vi "Parse Time.vi"(7 "Time In":T1, 10 "Time Index":i32, 11 "Fields In":string[](array[string])) -> (3 "Fields":string[](array[string]), 5 "Time":T1)   [LabVIEW 2012, in "nmea.lvlib" / "nmea.lvclass"]
uses:
  nmea.lvclass
  <vilib>/Utility/miscctls.llb/LVDateTimeRec.ctl
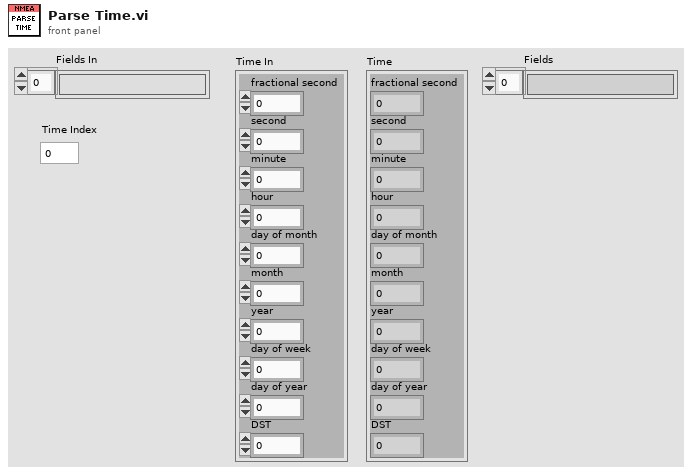
[diagram p1: front panel]
types:
  T1 = typedef "LVDateTimeRec.ctl" = cluster{"fractional second":dbl, "second":i32, "minute":i32, "hour":i32, "day of month":i32, "month":i32, "year":i32, "day of week":i32, "day of year":i32, "DST":i32}
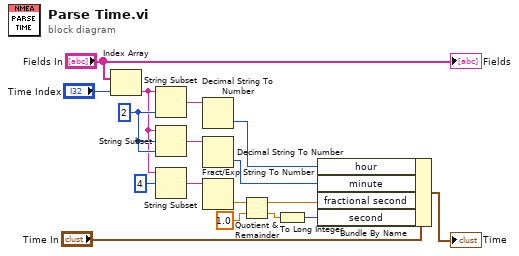
[diagram p0: block diagram]
diagram:
  w16 = 2 ("length (rest)")
  n1 = Index Array(array="Fields In", index="Time Index") -> (element=w15:string)
  n2 = String Subset(string=w15, length (rest)=w16) -> (substring=w11:string)  [unwired: 1 in]
  n3 = String Subset(string=w15, offset (0)=w16, length (rest)=w16) -> (substring=w12:string)
  n4 = String Subset(string=w15, offset (0)=4) -> (substring=w13:string)  [unwired: 1 in]
  n5 = Decimal String To Number(string=w11) -> (number=w2:i32)  [unwired: 2 in, 1 out]
  n6 = Decimal String To Number(string=w12) -> (number=w3:i32)  [unwired: 2 in, 1 out]
  n7 = Fract/Exp String To Number(string=w13) -> (number=w9:dbl)  [unwired: 3 in, 1 out]
  n8 = Quotient & Remainder(x=w9, y=1.0) -> (x-y*floor(x/y)=w6:dbl, floor(x/y)=w5:dbl)
  n9 = To Long Integer(number=w5) -> (32bit integer=w4:i32)
  n10 = Bundle By Name(cluster="Time In", "hour"=w2, "minute"=w3, "fractional second"=w6, "second"=w4) -> (→"Time":T1)
  "Fields" <- "Fields In"
